vi "main.vi"() -> ()   [LabVIEW 2012]
uses:
  <vilib>/Instr/_visa.llb/VISA Configure Serial Port (Instr).vi
panel:
  in  "VISA":refnum<visa-resource-name>="COM6"
  in  "退出":bool
  in  "系统设置":bool
  in  "病例管理":bool
  in  "创建用户":bool
  in  "震动4":enum32{"选项卡 1", "选项卡 2"}(tab)
  in  "震动3":enum32{"选项卡 1", "选项卡 2"}(tab)
  in  "震动2":enum32{"选项卡 1", "选项卡 2"}(tab)
  in  "震动1":enum32{"选项卡 1", "选项卡 2"}(tab)
  in  "定频 4":T1=1 items=["定频1"=1, "定频2"=2, "定频3"=3, "定频4"=4, "定频5"=5, "定频6"=6, "定频7"=7, "定频8"=8, "定频9"=9]
  in  "变频 4":T2=1 items=["变频1"=1, "变频2"=2, "变频3"=3, "变频4"=4, "变频5"=5, "变频6"=6, "变频7"=7, "变频8"=8, "变频9"=9, "变频10"=10, "变频11"=11]
  in  "输出 4":T3
  in  "停止 4":T4
  in  "震动 4":T5
  in  "档位 4":T6
  in  "定时 4":T7=1800 items=["5分钟"=300, "10分钟"=600, "20分钟"=1200, "30分钟"=1800, "60分钟"=3600, "90分钟"=5400, "120分钟"=7200, "180分钟"=10800]
  out "time 4":T8
  in  "定频 3":T1=1 items=["定频1"=1, "定频2"=2, "定频3"=3, "定频4"=4, "定频5"=5, "定频6"=6, "定频7"=7, "定频8"=8, "定频9"=9]
  in  "变频 3":T2=1 items=["变频1"=1, "变频2"=2, "变频3"=3, "变频4"=4, "变频5"=5, "变频6"=6, "变频7"=7, "变频8"=8, "变频9"=9, "变频10"=10, "变频11"=11]
  in  "输出 3":T3
  in  "停止 3":T4
  in  "震动 3":T5
  in  "档位 3":T6
  in  "定时 3":T7=1800 items=["5分钟"=300, "10分钟"=600, "20分钟"=1200, "30分钟"=1800, "60分钟"=3600, "90分钟"=5400, "120分钟"=7200, "180分钟"=10800]
  out "time 3":T8
  in  "定频 2":T1=1 items=["定频1"=1, "定频2"=2, "定频3"=3, "定频4"=4, "定频5"=5, "定频6"=6, "定频7"=7, "定频8"=8, "定频9"=9]
  in  "变频 2":T2=1 items=["变频1"=1, "变频2"=2, "变频3"=3, "变频4"=4, "变频5"=5, "变频6"=6, "变频7"=7, "变频8"=8, "变频9"=9, "变频10"=10, "变频11"=11]
  in  "输出 2":T3
  in  "停止 2":T4
  in  "震动 2":T5
  in  "档位 2":T6
  in  "定时 2":T7=1800 items=["5分钟"=300, "10分钟"=600, "20分钟"=1200, "30分钟"=1800, "60分钟"=3600, "90分钟"=5400, "120分钟"=7200, "180分钟"=10800]
  out "time 2":T8
  in  "定频 1":T1=1 items=["定频1"=1, "定频2"=2, "定频3"=3, "定频4"=4, "定频5"=5, "定频6"=6, "定频7"=7, "定频8"=8, "定频9"=9]
  in  "变频 1":T2=1 items=["变频1"=1, "变频2"=2, "变频3"=3, "变频4"=4, "变频5"=5, "变频6"=6, "变频7"=7, "变频8"=8, "变频9"=9, "变频10"=10, "变频11"=11]
  in  "输出 1":T3
  in  "停止 1":T4
  in  "震动 1":T5
  in  "档位 1":T6
  in  "定时 1":T7=1800 items=["5分钟"=300, "10分钟"=600, "20分钟"=1200, "30分钟"=1800, "60分钟"=3600, "90分钟"=5400, "120分钟"=7200, "180分钟"=10800]
  out "time 1":T8
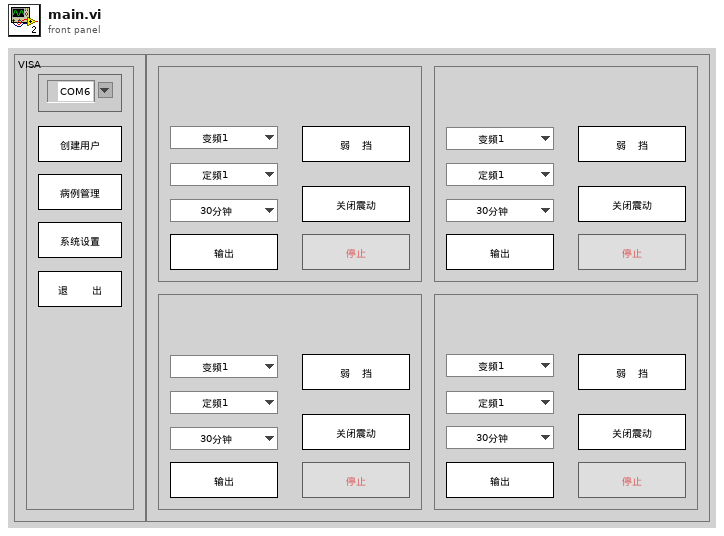
[diagram p1: front panel]
types:
  T1 = typedef "定频.ctl" = u8
  T2 = typedef "变频.ctl" = u8
  T3 = typedef "输出.ctl" = bool
  T4 = typedef "停止.ctl" = bool
  T5 = typedef "震动.ctl" = bool
  T6 = typedef "档位.ctl" = bool
  T7 = typedef "定时.ctl" = u16
  T8 = typedef "倒计时.ctl" = string
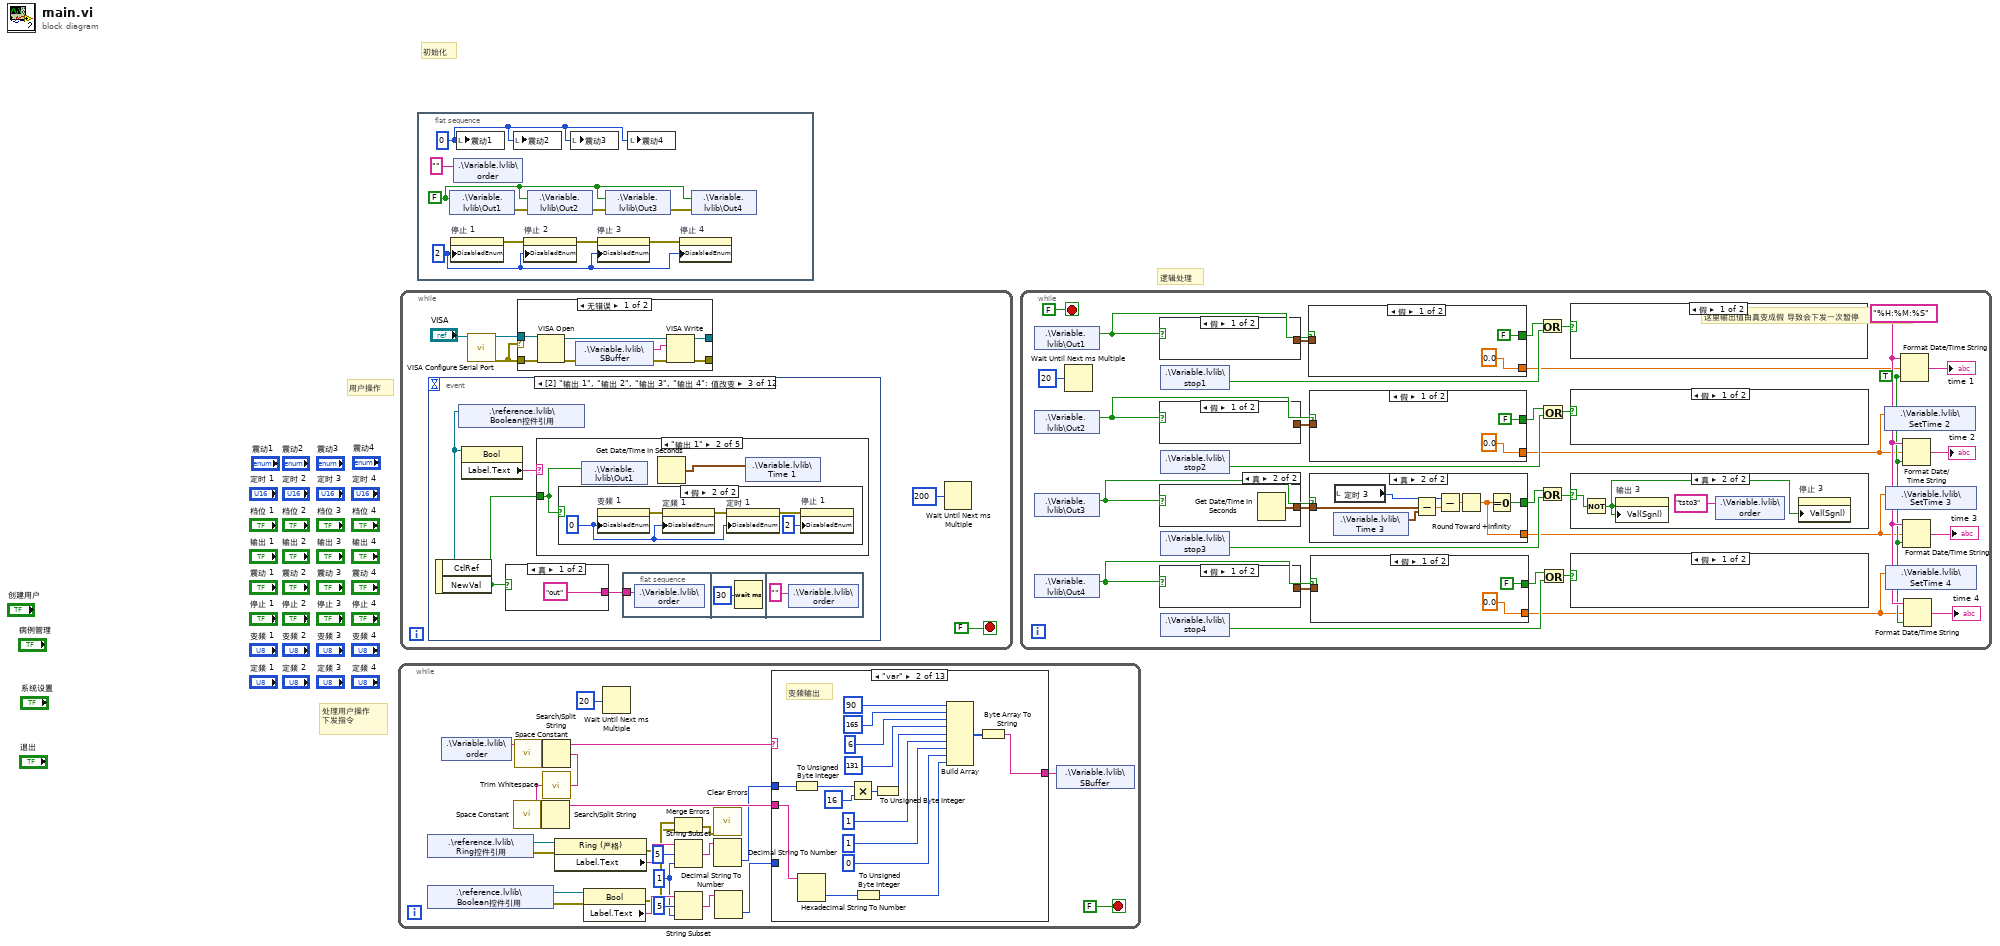
[diagram p0: block diagram]
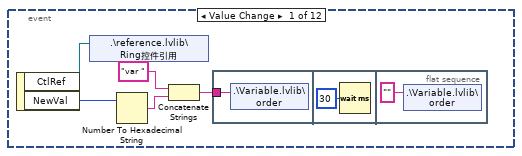
[diagram p3: hidden frame]
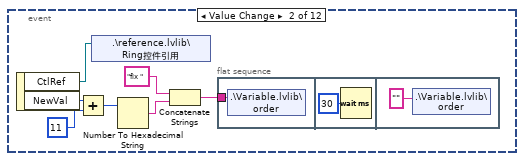
[diagram p4: hidden frame]
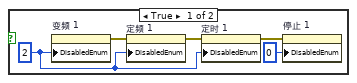
[diagram p6: hidden frame]
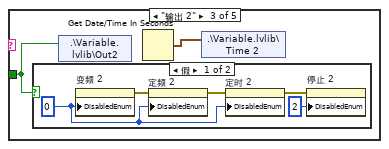
[diagram p7: hidden frame]
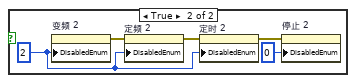
[diagram p8: hidden frame]
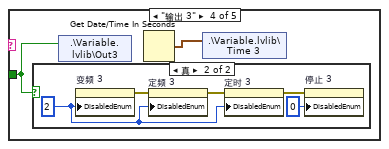
[diagram p9: hidden frame]
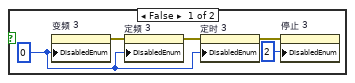
[diagram p10: hidden frame]
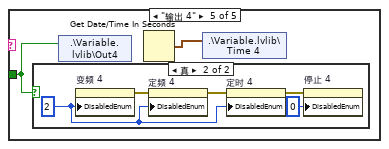
[diagram p11: hidden frame]
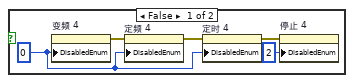
[diagram p12: hidden frame]
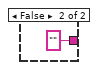
[diagram p13: hidden frame]
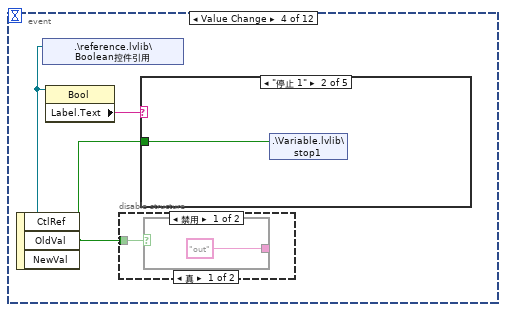
[diagram p14: hidden frame]
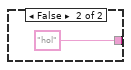
[diagram p15: hidden frame]
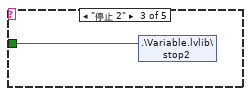
[diagram p18: hidden frame]
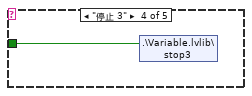
[diagram p19: hidden frame]
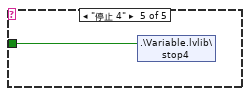
[diagram p20: hidden frame]
diagram:
  # "逻辑处理"
  # "处理用户操作\n下发指令"
  # "用户操作"
  # "初始化"
  # "这里输出值由真变成假 导致会下发一次暂停"
  n1 = while {
    stop <- FALSE stop-if-true
    w11 = 1
    n2 = shared-variable ".\\reference.lvlib\\Ring控件引用"() -> (w19:refnum<vi>, error out=w18:errorcluster)  [unwired: 1 in]
    n3 = shared-variable ".\\reference.lvlib\\Boolean控件引用"() -> (w17:refnum<vi>, error out=w16:errorcluster)  [unwired: 1 in]
    n4 = shared-variable ".\\Variable.lvlib\\order"() -> (w22:string)  [unwired: 1 in, 1 out]
    n5 = call <vilib>:"Space Constant.vi"() -> ("String"=w24:string)
    n6 = call <vilib>:"Space Constant.vi"() -> ("String"=w26:string)
    n7 = Search/Split String(string=w22, search string/char (-)=w26) -> (substring before match=w25:string, match + rest of string=w21:string)  [unwired: 1 in, 1 out]
    n8 = call <vilib>:"Trim Whitespace.vi"("string"=w21) -> ("trimmed string"=w20:string)  [unwired: 1 in]
    n9 = Search/Split String(string=w20, search string/char (-)=w24) -> (substring before match=w23:string)  [unwired: 1 in, 2 out]
    n10 = property class="Ring (严格)"(reference=w19, error in=w18) -> (error out=w5:errorcluster, "Label.Text"=w15:string)  [unwired: 1 out]
    n11 = property class="Bool"(reference=w17, error in=w16) -> (error out=w4:errorcluster, "Label.Text"=w13:string)  [unwired: 1 out]
    n12 = Wait Until Next ms Multiple(millisecond multiple=u32 20 ("毫秒倍数")) -> ()  [unwired: 1 out]
    n13 = Merge Errors(w5, w4) -> (w6:errorcluster)
    n14 = String Subset(string=w15, offset (0)=5 ("偏移量(0)"), length (rest)=w11) -> (substring=w10:string)
    n15 = String Subset(string=w13, offset (0)=5 ("偏移量(0)"), length (rest)=w11) -> (substring=w9:string)
    n16 = call <vilib>:"Clear Errors.vi"("error in (no error)"=w6) -> ()  [unwired: 6 in, 1 out]
    n17 = Decimal String To Number(string=w10) -> (number=w8:i32)  [unwired: 2 in, 1 out]
    n18 = Decimal String To Number(string=w9) -> (number=w7:i32)  [unwired: 2 in, 1 out]
    n19 = case shown="\"var\"" w25 {
      tunnel: w23 -> [_ w44 w61 _ _ _ _ _ _ _ _ _ _]
      tunnel: ["" ("string") w28 w45 w62 w77 w92 w106 w120 w134 w149 w168 w186 w201] -> w3
      tunnel: w8 -> [_ w30 w47 _ _ _ _ _ _ _ _ _ _]
      tunnel: w7 -> [_ _ _ w64 w79 _ _ _ _ w148 w167 w188 w203]
      frame Default {
      }
      frame "var" {
        # "变频输出"
        n20 = To Unsigned Byte Integer(number=w30) -> (unsigned 8bit integer=w29:u8)
        n21 = Hexadecimal String To Number(string=w44) -> (number=w36:u32)  [unwired: 2 in, 1 out]
        n22 = Multiply(x=w29, y=u8 16) -> (x*y=w37:u8)
        n23 = To Unsigned Byte Integer(number=w36) -> (unsigned 8bit integer=w31:u8)
        n24 = To Unsigned Byte Integer(number=w37) -> (unsigned 8bit integer=w35:u8)
        n25 = Build Array(u8 90, u8 165, u8 6, u8 131, w35, u8 1, u8 1, u8 0, w31) -> (w42:u8[])
        n26 = Byte Array To String(unsigned byte array=w42) -> (string=w28:string)
      }
      frame "fix" {
        # "定频输出"
        n27 = To Unsigned Byte Integer(number=w47) -> (unsigned 8bit integer=w46:u8)
        n28 = Hexadecimal String To Number(string=w61) -> (number=w53:u32)  [unwired: 2 in, 1 out]
        n29 = Multiply(x=w46, y=u8 16) -> (x*y=w54:u8)
        n30 = To Unsigned Byte Integer(number=w53) -> (unsigned 8bit integer=w48:u8)
        n31 = To Unsigned Byte Integer(number=w54) -> (unsigned 8bit integer=w52:u8)
        n32 = Build Array(u8 90, u8 165, u8 6, u8 131, w52, u8 1, u8 1, u8 0, w48) -> (w59:u8[])
        n33 = Byte Array To String(unsigned byte array=w59) -> (string=w45:string)
      }
      frame "out" {
        # "输出"
        n34 = To Unsigned Byte Integer(number=w64) -> (unsigned 8bit integer=w63:u8)
        n35 = Multiply(x=w63, y=u8 16) -> (x*y=w70:u8)
        n36 = To Unsigned Byte Integer(number=w70) -> (unsigned 8bit integer=w69:u8)
        n37 = Build Array(u8 90, u8 165, u8 6, u8 131, w69, u8 0, u8 1, u8 0, u8 1) -> (w75:u8[])
        n38 = Byte Array To String(unsigned byte array=w75) -> (string=w62:string)
      }
      frame "sto" {
        n39 = To Unsigned Byte Integer(number=w79) -> (unsigned 8bit integer=w78:u8)
        n40 = Multiply(x=w78, y=u8 16) -> (x*y=w85:u8)
        n41 = To Unsigned Byte Integer(number=w85) -> (unsigned 8bit integer=w84:u8)
        n42 = Build Array(u8 90, u8 165, u8 6, u8 131, w84, u8 0, u8 1, u8 0, u8 0) -> (w90:u8[])
        n43 = Byte Array To String(unsigned byte array=w90) -> (string=w77:string)
      }
      frame "tsto1" {
        n44 = Multiply(x=u8 1, y=u8 16) -> (x*y=w99:u8)
        n45 = To Unsigned Byte Integer(number=w99) -> (unsigned 8bit integer=w98:u8)
        n46 = Build Array(u8 90, u8 165, u8 6, u8 131, w98, u8 0, u8 1, u8 0, u8 0) -> (w104:u8[])
        n47 = Byte Array To String(unsigned byte array=w104) -> (string=w92:string)
      }
      frame "tsto2" {
        n48 = Multiply(x=u8 2, y=u8 16) -> (x*y=w113:u8)
        n49 = To Unsigned Byte Integer(number=w113) -> (unsigned 8bit integer=w112:u8)
        n50 = Build Array(u8 90, u8 165, u8 6, u8 131, w112, u8 0, u8 1, u8 0, u8 0) -> (w118:u8[])
        n51 = Byte Array To String(unsigned byte array=w118) -> (string=w106:string)
      }
      frame "tsto3" {
        n52 = Multiply(x=u8 3, y=u8 16) -> (x*y=w127:u8)
        n53 = To Unsigned Byte Integer(number=w127) -> (unsigned 8bit integer=w126:u8)
        n54 = Build Array(u8 90, u8 165, u8 6, u8 131, w126, u8 0, u8 1, u8 0, u8 0) -> (w132:u8[])
        n55 = Byte Array To String(unsigned byte array=w132) -> (string=w120:string)
      }
      frame "tsto4" {
        n56 = Multiply(x=u8 4, y=u8 16) -> (x*y=w141:u8)
        n57 = To Unsigned Byte Integer(number=w141) -> (unsigned 8bit integer=w140:u8)
        n58 = Build Array(u8 90, u8 165, u8 6, u8 131, w140, u8 0, u8 1, u8 0, u8 0) -> (w146:u8[])
        n59 = Byte Array To String(unsigned byte array=w146) -> (string=w134:string)
      }
      frame "sha" {
        n60 = To Unsigned Byte Integer(number=w148) -> (unsigned 8bit integer=w150:u8)
        n61 = Multiply(x=w150, y=u8 16) -> (x*y=w156:u8)
        n62 = To Unsigned Byte Integer(number=w156) -> (unsigned 8bit integer=w155:u8)
        n63 = Build Array(u8 90, u8 165, u8 6, u8 131, w155, u8 6, u8 1, u8 0, u8 1) -> (w161:u8[])
        n64 = case shown="4" w148 {
          frame 0, Default {
          }
          frame 1 {
            n65 = local write "震动1"(0) -> ()
          }
          frame 2 {
            n66 = local write "震动2"(0) -> ()
          }
          frame 3 {
            n67 = local write "震动3"(0) -> ()
          }
          frame 4 {
            n68 = local write "震动4"(0) -> ()
          }
        }
        n69 = Byte Array To String(unsigned byte array=w161) -> (string=w149:string)
      }
      frame "sth" {
        n70 = To Unsigned Byte Integer(number=w167) -> (unsigned 8bit integer=w169:u8)
        n71 = Multiply(x=w169, y=u8 16) -> (x*y=w175:u8)
        n72 = To Unsigned Byte Integer(number=w175) -> (unsigned 8bit integer=w174:u8)
        n73 = Build Array(u8 90, u8 165, u8 6, u8 131, w174, u8 6, u8 1, u8 0, u8 0) -> (w180:u8[])
        n74 = case shown="0, 默认" w167 {
          frame 0, Default {
          }
          frame 1 {
            n75 = local write "震动1"(1) -> ()
          }
          frame 2 {
            n76 = local write "震动2"(1) -> ()
          }
          frame 3 {
            n77 = local write "震动3"(1) -> ()
          }
          frame 4 {
            n78 = local write "震动4"(1) -> ()
          }
        }
        n79 = Byte Array To String(unsigned byte array=w180) -> (string=w168:string)
      }
      frame "pw1" {
        n80 = To Unsigned Byte Integer(number=w188) -> (unsigned 8bit integer=w187:u8)
        n81 = Multiply(x=w187, y=u8 16) -> (x*y=w194:u8)
        n82 = To Unsigned Byte Integer(number=w194) -> (unsigned 8bit integer=w193:u8)
        n83 = Build Array(u8 90, u8 165, u8 6, u8 131, w193, u8 5, u8 1, u8 0, u8 0) -> (w199:u8[])
        n84 = Byte Array To String(unsigned byte array=w199) -> (string=w186:string)
      }
      frame "pw2" {
        n85 = To Unsigned Byte Integer(number=w203) -> (unsigned 8bit integer=w202:u8)
        n86 = Multiply(x=w202, y=u8 16) -> (x*y=w209:u8)
        n87 = To Unsigned Byte Integer(number=w209) -> (unsigned 8bit integer=w208:u8)
        n88 = Build Array(u8 90, u8 165, u8 6, u8 131, w208, u8 5, u8 1, u8 0, u8 1) -> (w214:u8[])
        n89 = Byte Array To String(unsigned byte array=w214) -> (string=w201:string)
      }
    }
    n90 = shared-variable ".\\Variable.lvlib\\SBuffer"(w3) -> ()  [unwired: 1 in, 1 out]
  }
  n91 = while {
    stop <- FALSE stop-if-true
    n92 = event shown="[2] \"输出 1\", \"输出 2\", \"输出 3\", \"输出 4\": 值改变" {
      selector: _ -> [_ _ _ _ _ _ _ _ _ _ _ _]
      dyn-events: _ -> [_ _ _ _ _ _ _ _ _ _ _ _]
      timeout: _ -> [_ _ _ _ _ _ _ _ _ _ _ _]
      event Value Change {
        n93 = event-data() -> ("CtlRef"=w232:refnum<vi>, "NewVal"=w233:T2)  [unwired: 1 in]
        n94 = shared-variable ".\\reference.lvlib\\Ring控件引用"(w232) -> ()  [unwired: 1 in, 1 out]
        n95 = Number To Hexadecimal String(2:w233) -> (0:w235:string)  [unwired: 1 in]
        n96 = Concatenate Strings("var " ("字符串"), w235) -> (w231:string)
        n97 = flat-sequence {
          tunnel: w231 -> [w236]
          frame #0 {
            n98 = shared-variable ".\\Variable.lvlib\\order"(w236) -> ()  [unwired: 1 in, 1 out]
          }
          frame #1 {
            n99 = Wait (ms)(milliseconds to wait=u32 30 ("等待时间（毫秒）")) -> ()  [unwired: 1 out]
          }
          frame #2 {
            n100 = shared-variable ".\\Variable.lvlib\\order"("" ("order")) -> ()  [unwired: 1 in, 1 out]
          }
        }
      }
      event Value Change {
        n101 = event-data() -> ("CtlRef"=w240:refnum<vi>, "NewVal"=w242:T1)  [unwired: 1 in]
        n102 = Add(x=w242, y=11) -> (x+y=w243:i32)
        n103 = shared-variable ".\\reference.lvlib\\Ring控件引用"(w240) -> ()  [unwired: 1 in, 1 out]
        n104 = Number To Hexadecimal String(2:w243) -> (0:w245:string)  [unwired: 1 in]
        n105 = Concatenate Strings("fix " ("字符串"), w245) -> (w239:string)
        n106 = flat-sequence {
          tunnel: w239 -> [w246]
          frame #0 {
            n107 = shared-variable ".\\Variable.lvlib\\order"(w246) -> ()  [unwired: 1 in, 1 out]
          }
          frame #1 {
            n108 = Wait (ms)(milliseconds to wait=u32 30 ("等待时间（毫秒）")) -> ()  [unwired: 1 out]
          }
          frame #2 {
            n109 = shared-variable ".\\Variable.lvlib\\order"("" ("order")) -> ()  [unwired: 1 in, 1 out]
          }
        }
      }
      event Value Change {
        n110 = event-data() -> ("CtlRef"=w250:refnum<vi>, "NewVal"=w251:T3)  [unwired: 1 in]
        n111 = shared-variable ".\\reference.lvlib\\Boolean控件引用"(w250) -> ()  [unwired: 1 in, 1 out]
        n112 = property class="Bool"(reference=w250) -> ("Label.Text"=w252:string)  [unwired: 1 in, 2 out]
        n113 = case shown="真" w251 {
          tunnel: ["out" ""] -> w249
          frame True {
          }
          frame False {
          }
        }
        n114 = case shown="\"输出 1\"" w252 {
          tunnel: w251 -> [_ w257 w269 w281 w293]
          frame "假", Default {
          }
          frame "输出 1" {
            n115 = case shown="假" w257 {
              frame True {
                w259 = 2
                n116 = property on="变频 1" class="Ring (严格)"("DisabledEnum"=w259) -> (error out=w262:errorcluster)  [unwired: 2 in, 1 out]
                n117 = property on="定频 1" class="Ring (严格)"(error in=w262, "DisabledEnum"=w259) -> (error out=w261:errorcluster)  [unwired: 1 in, 1 out]
                n118 = property on="定时 1" class="Ring (严格)"(error in=w261, "DisabledEnum"=w259) -> (error out=w260:errorcluster)  [unwired: 1 in, 1 out]
                n119 = property on="停止 1" class="Bool"(error in=w260, "DisabledEnum"=0) -> ()  [unwired: 1 in, 2 out]
              }
              frame False {
                w264 = 0
                n120 = property on="变频 1" class="Ring (严格)"("DisabledEnum"=w264) -> (error out=w267:errorcluster)  [unwired: 2 in, 1 out]
                n121 = property on="定频 1" class="Ring (严格)"(error in=w267, "DisabledEnum"=w264) -> (error out=w266:errorcluster)  [unwired: 1 in, 1 out]
                n122 = property on="定时 1" class="Ring (严格)"(error in=w266, "DisabledEnum"=w264) -> (error out=w265:errorcluster)  [unwired: 1 in, 1 out]
                n123 = property on="停止 1" class="Bool"(error in=w265, "DisabledEnum"=2) -> ()  [unwired: 1 in, 2 out]
              }
            }
            n124 = shared-variable ".\\Variable.lvlib\\Out1"(w257) -> ()  [unwired: 1 in, 1 out]
            n125 = Get Date/Time In Seconds() -> (seconds since 1Jan1904=w256:timestamp)
            n126 = shared-variable ".\\Variable.lvlib\\Time 1"(w256) -> ()  [unwired: 1 in, 1 out]
          }
          frame "输出 2" {
            n127 = case shown="假" w269 {
              frame False {
                w271 = 0
                n128 = property on="变频 2" class="Ring (严格)"("DisabledEnum"=w271) -> (error out=w274:errorcluster)  [unwired: 2 in, 1 out]
                n129 = property on="定频 2" class="Ring (严格)"(error in=w274, "DisabledEnum"=w271) -> (error out=w273:errorcluster)  [unwired: 1 in, 1 out]
                n130 = property on="定时 2" class="Ring (严格)"(error in=w273, "DisabledEnum"=w271) -> (error out=w272:errorcluster)  [unwired: 1 in, 1 out]
                n131 = property on="停止 2" class="Bool"(error in=w272, "DisabledEnum"=2) -> ()  [unwired: 1 in, 2 out]
              }
              frame True {
                w276 = 2
                n132 = property on="变频 2" class="Ring (严格)"("DisabledEnum"=w276) -> (error out=w279:errorcluster)  [unwired: 2 in, 1 out]
                n133 = property on="定频 2" class="Ring (严格)"(error in=w279, "DisabledEnum"=w276) -> (error out=w278:errorcluster)  [unwired: 1 in, 1 out]
                n134 = property on="定时 2" class="Ring (严格)"(error in=w278, "DisabledEnum"=w276) -> (error out=w277:errorcluster)  [unwired: 1 in, 1 out]
                n135 = property on="停止 2" class="Bool"(error in=w277, "DisabledEnum"=0) -> ()  [unwired: 1 in, 2 out]
              }
            }
            n136 = shared-variable ".\\Variable.lvlib\\Out2"(w269) -> ()  [unwired: 1 in, 1 out]
            n137 = Get Date/Time In Seconds() -> (seconds since 1Jan1904=w268:timestamp)
            n138 = shared-variable ".\\Variable.lvlib\\Time 2"(w268) -> ()  [unwired: 1 in, 1 out]
          }
          frame "输出 3" {
            n139 = case shown="真" w281 {
              frame False {
                w283 = 0
                n140 = property on="变频 3" class="Ring (严格)"("DisabledEnum"=w283) -> (error out=w286:errorcluster)  [unwired: 2 in, 1 out]
                n141 = property on="定频 3" class="Ring (严格)"(error in=w286, "DisabledEnum"=w283) -> (error out=w285:errorcluster)  [unwired: 1 in, 1 out]
                n142 = property on="定时 3" class="Ring (严格)"(error in=w285, "DisabledEnum"=w283) -> (error out=w284:errorcluster)  [unwired: 1 in, 1 out]
                n143 = property on="停止 3" class="Bool"(error in=w284, "DisabledEnum"=2) -> ()  [unwired: 1 in, 2 out]
              }
              frame True {
                w288 = 2
                n144 = property on="变频 3" class="Ring (严格)"("DisabledEnum"=w288) -> (error out=w291:errorcluster)  [unwired: 2 in, 1 out]
                n145 = property on="定频 3" class="Ring (严格)"(error in=w291, "DisabledEnum"=w288) -> (error out=w290:errorcluster)  [unwired: 1 in, 1 out]
                n146 = property on="定时 3" class="Ring (严格)"(error in=w290, "DisabledEnum"=w288) -> (error out=w289:errorcluster)  [unwired: 1 in, 1 out]
                n147 = property on="停止 3" class="Bool"(error in=w289, "DisabledEnum"=0) -> ()  [unwired: 1 in, 2 out]
              }
            }
            n148 = shared-variable ".\\Variable.lvlib\\Out3"(w281) -> ()  [unwired: 1 in, 1 out]
            n149 = Get Date/Time In Seconds() -> (seconds since 1Jan1904=w280:timestamp)
            n150 = shared-variable ".\\Variable.lvlib\\Time 3"(w280) -> ()  [unwired: 1 in, 1 out]
          }
          frame "输出 4" {
            n151 = case shown="真" w293 {
              frame False {
                w295 = 0
                n152 = property on="变频 4" class="Ring (严格)"("DisabledEnum"=w295) -> (error out=w298:errorcluster)  [unwired: 2 in, 1 out]
                n153 = property on="定频 4" class="Ring (严格)"(error in=w298, "DisabledEnum"=w295) -> (error out=w297:errorcluster)  [unwired: 1 in, 1 out]
                n154 = property on="定时 4" class="Ring (严格)"(error in=w297, "DisabledEnum"=w295) -> (error out=w296:errorcluster)  [unwired: 1 in, 1 out]
                n155 = property on="停止 4" class="Bool"(error in=w296, "DisabledEnum"=2) -> ()  [unwired: 1 in, 2 out]
              }
              frame True {
                w300 = 2
                n156 = property on="变频 4" class="Ring (严格)"("DisabledEnum"=w300) -> (error out=w303:errorcluster)  [unwired: 2 in, 1 out]
                n157 = property on="定频 4" class="Ring (严格)"(error in=w303, "DisabledEnum"=w300) -> (error out=w302:errorcluster)  [unwired: 1 in, 1 out]
                n158 = property on="定时 4" class="Ring (严格)"(error in=w302, "DisabledEnum"=w300) -> (error out=w301:errorcluster)  [unwired: 1 in, 1 out]
                n159 = property on="停止 4" class="Bool"(error in=w301, "DisabledEnum"=0) -> ()  [unwired: 1 in, 2 out]
              }
            }
            n160 = shared-variable ".\\Variable.lvlib\\Out4"(w293) -> ()  [unwired: 1 in, 1 out]
            n161 = Get Date/Time In Seconds() -> (seconds since 1Jan1904=w292:timestamp)
            n162 = shared-variable ".\\Variable.lvlib\\Time 4"(w292) -> ()  [unwired: 1 in, 1 out]
          }
        }
        n163 = flat-sequence {
          tunnel: w249 -> [w253]
          frame #0 {
            n164 = shared-variable ".\\Variable.lvlib\\order"(w253) -> ()  [unwired: 1 in, 1 out]
          }
          frame #1 {
            n165 = Wait (ms)(milliseconds to wait=u32 30 ("等待时间（毫秒）")) -> ()  [unwired: 1 out]
          }
          frame #2 {
            n166 = shared-variable ".\\Variable.lvlib\\order"("" ("order")) -> ()  [unwired: 1 in, 1 out]
          }
        }
      }
      event Value Change {
        n167 = event-data() -> ("CtlRef"=w307:refnum<vi>, "NewVal"=w306:T4)  [unwired: 1 in, 1 out]
        n168 = shared-variable ".\\reference.lvlib\\Boolean控件引用"(w307) -> ()  [unwired: 1 in, 1 out]
        n169 = property class="Bool"(reference=w307) -> ("Label.Text"=w308:string)  [unwired: 1 in, 2 out]
        n170 = disable-structure shown="禁用" {
          disable-tunnel: w306 -> [w309 _]
          frame Disabled {
            n171 = case shown="真" w309 {
              tunnel: ["out" "hol"] -> _
              frame True {
              }
              frame False {
              }
            }
          }
          frame Enabled {
          }
        }
        n172 = case shown="\"停止 1\"" w308 {
          tunnel: w306 -> [_ w312 w313 w314 w315]
          frame "假", Default {
          }
          frame "停止 1" {
            n173 = shared-variable ".\\Variable.lvlib\\stop1"(w312) -> ()  [unwired: 1 in, 1 out]
          }
          frame "停止 2" {
            n174 = shared-variable ".\\Variable.lvlib\\stop2"(w313) -> ()  [unwired: 1 in, 1 out]
          }
          frame "停止 3" {
            n175 = shared-variable ".\\Variable.lvlib\\stop3"(w314) -> ()  [unwired: 1 in, 1 out]
          }
          frame "停止 4" {
            n176 = shared-variable ".\\Variable.lvlib\\stop4"(w315) -> ()  [unwired: 1 in, 1 out]
          }
        }
      }
      event Value Change {
        n177 = event-data() -> ("CtlRef"=w316:refnum<vi>, "NewVal"=w318:T5)  [unwired: 1 in]
        n178 = shared-variable ".\\reference.lvlib\\Boolean控件引用"(w316) -> ()  [unwired: 1 in, 1 out]
        n179 = case shown="真" w318 {
          tunnel: ["sth" "sha"] -> w317
          frame True {
          }
          frame False {
          }
        }
        n180 = flat-sequence {
          tunnel: w317 -> [w319]
          frame #0 {
            n181 = shared-variable ".\\Variable.lvlib\\order"(w319) -> ()  [unwired: 1 in, 1 out]
          }
          frame #1 {
            n182 = Wait (ms)(milliseconds to wait=u32 30 ("等待时间（毫秒）")) -> ()  [unwired: 1 out]
          }
          frame #2 {
            n183 = shared-variable ".\\Variable.lvlib\\order"("" ("order")) -> ()  [unwired: 1 in, 1 out]
          }
        }
      }
      event Value Change {
        n184 = event-data() -> ("CtlRef"=w325:refnum<vi>, "NewVal"=w326:T6)  [unwired: 1 in]
        n185 = shared-variable ".\\reference.lvlib\\Boolean控件引用"(w325) -> ()  [unwired: 1 in, 1 out]
        n186 = case shown="假" w326 {
          tunnel: ["pw2" "pw1"] -> w324
          frame True {
          }
          frame False {
          }
        }
        n187 = flat-sequence {
          tunnel: w324 -> [w327]
          frame #0 {
            n188 = shared-variable ".\\Variable.lvlib\\order"(w327) -> ()  [unwired: 1 in, 1 out]
          }
          frame #1 {
            n189 = Wait (ms)(milliseconds to wait=u32 30 ("等待时间（毫秒）")) -> ()  [unwired: 1 out]
          }
          frame #2 {
            n190 = shared-variable ".\\Variable.lvlib\\order"("" ("order")) -> ()  [unwired: 1 in, 1 out]
          }
        }
      }
      event "VISA": Value Change {
        n191 = event-data() -> ("OldVal"=w335:refnum<visa-resource-name>, "NewVal"=w334:refnum<visa-resource-name>)  [unwired: 1 in]
        n192 = VISA Close(VISA resource name=w335) -> (error out=w333:errorcluster)  [unwired: 1 in]
        n193 = VISA Open(error in (no error)=w333, VISA resource name=w334) -> (error out=w332:errorcluster)  [unwired: 3 in, 1 out]
        n194 = call <vilib>:"General Error Handler.vi"("error in (no error)"=w332) -> ()  [unwired: 10 in, 5 out]
      }
      event Panel Close? {
        n195 = event-data() -> ()  [unwired: 1 in, 1 out]
        n196 = shared-variable ".\\Variable.lvlib\\Out4"() -> (w338:bool)  [unwired: 1 in, 1 out]
        n197 = shared-variable ".\\Variable.lvlib\\Out3"() -> (w339:bool)  [unwired: 1 in, 1 out]
        n198 = shared-variable ".\\Variable.lvlib\\Out1"() -> (w340:bool)  [unwired: 1 in, 1 out]
        n199 = shared-variable ".\\Variable.lvlib\\Out2"() -> (w341:bool)  [unwired: 1 in, 1 out]
        n200 = Compound Arithmetic op=OR(w340, w341, w339, w338) -> (w337:bool)
        n201 = case shown="假" w337 {
          tunnel: [w342 w345] -> w336
          frame True {
            n202 = Two Button Dialog(message="正在治疗中！！   \n请确认是否关闭" ("消息")) -> (T button?=w343:bool)  [unwired: 2 in]
            n203 = Not(x=w343) -> (.not. x?=w342:bool)
          }
          frame False {
            n204 = Two Button Dialog(message="软件即将关闭！" ("消息")) -> (T button?=w346:bool)  [unwired: 2 in]
            n205 = Not(x=w346) -> (.not. x?=w345:bool)
          }
        }
        n206 = event-data("Discard?"=w336) -> ()  [unwired: 1 in, 1 out]
      }
      event "退出": Value Change {
        n207 = event-data() -> ()  [unwired: 1 in, 3 out]
        n208 = shared-variable ".\\Variable.lvlib\\Out4"() -> (w350:bool)  [unwired: 1 in, 1 out]
        n209 = shared-variable ".\\Variable.lvlib\\Out3"() -> (w351:bool)  [unwired: 1 in, 1 out]
        n210 = shared-variable ".\\Variable.lvlib\\Out1"() -> (w352:bool)  [unwired: 1 in, 1 out]
        n211 = shared-variable ".\\Variable.lvlib\\Out2"() -> (w353:bool)  [unwired: 1 in, 1 out]
        n212 = Compound Arithmetic op=OR(w352, w353, w351, w350) -> (w349:bool)
        n213 = case shown="假" w349 {
          tunnel: [w355 w358] -> w348
          frame True {
            n214 = Two Button Dialog(message="正在治疗中！！   \n请确认是否关闭" ("消息")) -> (T button?=w356:bool)  [unwired: 2 in]
            n215 = Not(x=w356) -> (.not. x?=w355:bool)
          }
          frame False {
            n216 = Two Button Dialog(message="软件即将关闭！" ("消息")) -> (T button?=w358:bool)  [unwired: 2 in]
          }
        }
        n217 = case shown="真" w348 {
          frame False {
          }
          frame True {
            n218 = local read "VISA"() -> (w354:refnum<visa-resource-name>)
            n219 = VISA Close(VISA resource name=w354) -> ()  [unwired: 1 in, 1 out]
          }
        }
        n220 = Quit LabVIEW(quit? (T)=w348) -> ()
      }
      event "创建用户": Value Change {
        n221 = event-data() -> ()  [unwired: 1 in, 3 out]
        n222 = Current VI's Path() -> (path=w370:path)
        n223 = Build Path(base path=w370, name or relative path="..\\SubVIs\\adduser.vi" ("名称或相对路径")) -> (appended path=w371:path)
        n224 = Open VI Reference(vi path=w371) -> (vi reference=w368:refnum<vi>, error out=w367:errorcluster)  [unwired: 5 in]
        n225 = invoke class="VI" method="Run VI"(reference=w368, error in=w367, "Wait until done"=FALSE ("结束前等待"), "Auto Dispose Ref"=FALSE ("自动销毁引用")) -> (reference out=w364:refnum<vi>, error out=w363:errorcluster)  [unwired: 1 in, 3 out]
        n226 = invoke class="VI" method="FP.Open"(reference=w364, error in=w363, "Activate"=TRUE ("激活？")) -> (reference out=w360:refnum<vi>, error out=w361:errorcluster)  [unwired: 2 in, 3 out]
        n227 = Close Reference(reference=w360, error in (no error)=w361) -> ()  [unwired: 1 out]
      }
      event "病例管理": Value Change {
        n228 = event-data() -> ()  [unwired: 1 in, 3 out]
        n229 = Current VI's Path() -> (path=w383:path)
        n230 = Build Path(base path=w383, name or relative path="..\\SubVIs\\PatManage.vi" ("名称或相对路径")) -> (appended path=w384:path)
        n231 = Open VI Reference(vi path=w384) -> (vi reference=w381:refnum<vi>, error out=w380:errorcluster)  [unwired: 5 in]
        n232 = invoke class="VI" method="Run VI"(reference=w381, error in=w380, "Wait until done"=FALSE ("结束前等待"), "Auto Dispose Ref"=FALSE ("自动销毁引用")) -> (reference out=w377:refnum<vi>, error out=w376:errorcluster)  [unwired: 1 in, 3 out]
        n233 = invoke class="VI" method="FP.Open"(reference=w377, error in=w376, "Activate"=TRUE ("激活？")) -> (reference out=w373:refnum<vi>, error out=w374:errorcluster)  [unwired: 2 in, 3 out]
        n234 = Close Reference(reference=w373, error in (no error)=w374) -> (error out=w372:errorcluster)
        n235 = call <vilib>:"Clear Errors.vi"("error in (no error)"=w372) -> ()  [unwired: 6 in, 1 out]
      }
      event "系统设置": Value Change {
        n236 = event-data() -> ()  [unwired: 1 in, 3 out]
        n237 = call "医院信息设置"() -> ("联系电话"=w390:string, "联系人"=w391:string, "医院地址"=w392:string, "医院名称"=w393:string, "确定"=w385:bool)  [unwired: 14 in, 1 out]
        n238 = Current VI's Path() -> (path=w397:path)
        n239 = case shown="假" w385 {
          tunnel: w393 -> [_ w404]
          tunnel: w392 -> [_ w403]
          tunnel: w391 -> [_ w402]
          tunnel: w390 -> [_ w400]
          tunnel: [_ w399] -> w389
          frame False {
          }
          frame True {
            n240 = call <vilib>:"Space Constant.vi"() -> ("String"=w401:string)
            n241 = Concatenate Strings(w404, w401, w403, w401, w402, w401, w400) -> (w399:string)
          }
        }
        n242 = Build Path(base path=w397, name or relative path="..\\DATA\\HosInfor.txt" ("名称或相对路径")) -> (appended path=w398:path)
        n243 = Open/Create/Replace File(file path (use dialog)=w398) -> (refnum out=w394:refnum<file>, error out=w395:errorcluster)  [unwired: 5 in, 1 out]
        n244 = Write to Text File(file (use dialog)=w394, text=w389, error in=w395) -> (refnum out=w388:refnum<file>, error out=w386:errorcluster)  [unwired: 1 in, 1 out]
        n245 = case shown="真" w385 {
          tunnel: w386 -> [_ w405]
          frame False {
          }
          frame True {
            n246 = case shown="无错误" w405 {
              frame No Error {
                n247 = One Button Dialog(message="设置成功！" ("消息")) -> ()  [unwired: 1 in, 1 out]
              }
              frame Error {
              }
            }
          }
        }
        n248 = Close File(refnum=w388, error in=w386) -> (error out=w387:errorcluster)  [unwired: 1 out]
        n249 = call <vilib>:"General Error Handler.vi"("error in (no error)"=w387) -> ()  [unwired: 10 in, 5 out]
      }
    }
    n250 = call-poly "VISA Configure Serial Port"("VISA resource name"="VISA") -> ("VISA resource name out"=w219:refnum<visa-resource-name>, "error out"=w218:errorcluster)  [unwired: 13 in]
    n251 = case shown="无错误" w218 {
      tunnel: w219 -> [w223 w230]
      tunnel: w218 -> [w221 w229]
      tunnel: [w228 w229] -> _
      tunnel: [w227 w230] -> _
      frame No Error {
        n252 = VISA Open(error in (no error)=w221, VISA resource name=w223) -> (VISA resource name=w222:refnum<visa-resource-name>, error out=w224:errorcluster)  [unwired: 3 in]
        n253 = shared-variable ".\\Variable.lvlib\\SBuffer"(error in=w224) -> (w225:string, error out=w226:errorcluster)
        n254 = VISA Write(VISA resource name=w222, write buffer=w225, error in (no error)=w226) -> (VISA resource name out=w227:refnum<visa-resource-name>, error out=w228:errorcluster)  [unwired: 1 out]
      }
      frame Error {
      }
    }
    n255 = Wait Until Next ms Multiple(millisecond multiple=u32 200 ("毫秒倍数")) -> ()  [unwired: 1 out]
  }
  n256 = flat-sequence {
    frame #0 {
      w407 = 0
      w409 = FALSE ("Out1")
      w413 = 2
      n257 = shared-variable ".\\Variable.lvlib\\Out1"(w409) -> (error out=w412:errorcluster)  [unwired: 1 in]
      n258 = property on="停止 1" class="Bool"("DisabledEnum"=w413) -> (error out=w416:errorcluster)  [unwired: 2 in, 1 out]
      n259 = shared-variable ".\\Variable.lvlib\\order"("" ("发送")) -> ()  [unwired: 1 in, 1 out]
      n260 = local write "震动1"(w407) -> ()
      n261 = local write "震动2"(w407) -> ()
      n262 = property on="停止 2" class="Bool"(error in=w416, "DisabledEnum"=w413) -> (error out=w415:errorcluster)  [unwired: 1 in, 1 out]
      n263 = shared-variable ".\\Variable.lvlib\\Out2"(w409, error in=w412) -> (error out=w411:errorcluster)
      n264 = local write "震动3"(w407) -> ()
      n265 = property on="停止 3" class="Bool"(error in=w415, "DisabledEnum"=w413) -> (error out=w414:errorcluster)  [unwired: 1 in, 1 out]
      n266 = shared-variable ".\\Variable.lvlib\\Out3"(w409, error in=w411) -> (error out=w410:errorcluster)
      n267 = local write "震动4"(w407) -> ()
      n268 = property on="停止 4" class="Bool"(error in=w414, "DisabledEnum"=w413) -> ()  [unwired: 1 in, 2 out]
      n269 = shared-variable ".\\Variable.lvlib\\Out4"(w409, error in=w410) -> ()  [unwired: 1 out]
    }
  }
  n270 = while {
    stop <- FALSE stop-if-true
    w434 = TRUE ("UTC格式")
    w439 = "%H:%M:%S" ("时间格式字符串(%c)")
    n271 = shared-variable ".\\Variable.lvlib\\Out1"() -> (w443:bool)  [unwired: 1 in, 1 out]
    n272 = shared-variable ".\\Variable.lvlib\\Out2"() -> (w442:bool)  [unwired: 1 in, 1 out]
    n273 = shared-variable ".\\Variable.lvlib\\Out3"() -> (w441:bool)  [unwired: 1 in, 1 out]
    n274 = shared-variable ".\\Variable.lvlib\\Out4"() -> (w440:bool)  [unwired: 1 in, 1 out]
    n275 = Wait Until Next ms Multiple(millisecond multiple=u32 20 ("毫秒倍数")) -> ()  [unwired: 1 out]
    n276 = case shown="假" w443 {
      tunnel: [_ w500] -> w447
      frame False {
      }
      frame True {
        n277 = Get Date/Time In Seconds() -> (seconds since 1Jan1904=w500:timestamp)
      }
    }
    n278 = case shown="假" w442 {
      tunnel: [_ w499] -> w446
      frame False {
      }
      frame True {
        n279 = Get Date/Time In Seconds() -> (seconds since 1Jan1904=w499:timestamp)
      }
    }
    n280 = case shown="真" w441 {
      tunnel: [_ w498] -> w445
      frame False {
      }
      frame True {
        n281 = Get Date/Time In Seconds() -> (seconds since 1Jan1904=w498:timestamp)
      }
    }
    n282 = case shown="假" w440 {
      tunnel: [_ w497] -> w444
      frame False {
      }
      frame True {
        n283 = Get Date/Time In Seconds() -> (seconds since 1Jan1904=w497:timestamp)
      }
    }
    n284 = shared-variable ".\\Variable.lvlib\\stop1"() -> (w425:bool)  [unwired: 1 in, 1 out]
    n285 = shared-variable ".\\Variable.lvlib\\stop2"() -> (w424:bool)  [unwired: 1 in, 1 out]
    n286 = shared-variable ".\\Variable.lvlib\\stop3"() -> (w423:bool)  [unwired: 1 in, 1 out]
    n287 = shared-variable ".\\Variable.lvlib\\stop4"() -> (w422:bool)  [unwired: 1 in, 1 out]
    n288 = case shown="假" w443 {
      tunnel: w447 -> [_ w484]
      tunnel: [FALSE w480] -> w429
      tunnel: [0.0 w479] -> w421
      frame False {
      }
      frame True {
        n289 = shared-variable ".\\Variable.lvlib\\Time 1"() -> (w483:timestamp)  [unwired: 1 in, 1 out]
        n290 = local read "定时 1"() -> (w478:T7)
        n291 = Subtract(x=w484, y=w483) -> (x-y=w482:dbl)
        n292 = Subtract(x=w478, y=w482) -> (x-y=w481:dbl)
        n293 = Round Toward +Infinity(x=w481) -> (ceil(x): smallest int >= x=w479:dbl)
        n294 = Equal To 0?(x=w479) -> (x = 0?=w480:bool)
      }
    }
    n295 = case shown="假" w442 {
      tunnel: w446 -> [_ w472]
      tunnel: [FALSE w471] -> w428
      tunnel: [0.0 w470] -> w420
      frame False {
      }
      frame True {
        n296 = shared-variable ".\\Variable.lvlib\\Time 2"() -> (w474:timestamp)  [unwired: 1 in, 1 out]
        n297 = local read "定时 2"() -> (w469:T7)
        n298 = Subtract(x=w472, y=w474) -> (x-y=w475:dbl)
        n299 = Subtract(x=w469, y=w475) -> (x-y=w473:dbl)
        n300 = Round Toward +Infinity(x=w473) -> (ceil(x): smallest int >= x=w470:dbl)
        n301 = Equal To 0?(x=w470) -> (x = 0?=w471:bool)
      }
    }
    n302 = case shown="真" w441 {
      tunnel: w445 -> [_ w463]
      tunnel: [FALSE w462] -> w427
      tunnel: [0.0 w461] -> w419
      frame False {
      }
      frame True {
        n303 = shared-variable ".\\Variable.lvlib\\Time 3"() -> (w466:timestamp)  [unwired: 1 in, 1 out]
        n304 = local read "定时 3"() -> (w460:T7)
        n305 = Subtract(x=w463, y=w466) -> (x-y=w465:dbl)
        n306 = Subtract(x=w460, y=w465) -> (x-y=w464:dbl)
        n307 = Round Toward +Infinity(x=w464) -> (ceil(x): smallest int >= x=w461:dbl)
        n308 = Equal To 0?(x=w461) -> (x = 0?=w462:bool)
      }
    }
    n309 = case shown="假" w440 {
      tunnel: w444 -> [_ w454]
      tunnel: [FALSE w453] -> w426
      tunnel: [0.0 w452] -> w418
      frame False {
      }
      frame True {
        n310 = shared-variable ".\\Variable.lvlib\\Time 4"() -> (w456:timestamp)  [unwired: 1 in, 1 out]
        n311 = local read "定时 4"() -> (w451:T7)
        n312 = Subtract(x=w454, y=w456) -> (x-y=w457:dbl)
        n313 = Subtract(x=w451, y=w457) -> (x-y=w455:dbl)
        n314 = Round Toward +Infinity(x=w455) -> (ceil(x): smallest int >= x=w452:dbl)
        n315 = Equal To 0?(x=w452) -> (x = 0?=w453:bool)
      }
    }
    n316 = Or(x=w429, y=w425) -> (x .or. y?=w432:bool)
    n317 = Or(x=w427, y=w423) -> (x .or. y?=w431:bool)
    n318 = Or(x=w428, y=w424) -> (x .or. y?=w433:bool)
    n319 = Or(x=w426, y=w422) -> (x .or. y?=w430:bool)
    n320 = case shown="假" w432 {
      selector: w432 -> [_ w496]
      frame False {
      }
      frame True {
        n321 = Not(x=w496) -> (.not. x?=w494:bool)
        n322 = property on="输出 1" class="Bool"("Val(Sgnl)"=w494) -> ()  [unwired: 2 in, 2 out]
        n323 = shared-variable ".\\Variable.lvlib\\order"("tsto1" ("order")) -> ()  [unwired: 1 in, 1 out]
        n324 = property on="停止 1" class="Bool"("Val(Sgnl)"=w494) -> ()  [unwired: 2 in, 2 out]
      }
    }
    n325 = case shown="假" w433 {
      selector: w433 -> [_ w493]
      frame False {
      }
      frame True {
        n326 = Not(x=w493) -> (.not. x?=w491:bool)
        n327 = property on="输出 2" class="Bool"("Val(Sgnl)"=w491) -> ()  [unwired: 2 in, 2 out]
        n328 = shared-variable ".\\Variable.lvlib\\order"("tsto2" ("order")) -> ()  [unwired: 1 in, 1 out]
        n329 = property on="停止 2" class="Bool"("Val(Sgnl)"=w491) -> ()  [unwired: 2 in, 2 out]
      }
    }
    n330 = case shown="真" w431 {
      selector: w431 -> [_ w490]
      frame False {
      }
      frame True {
        n331 = Not(x=w490) -> (.not. x?=w488:bool)
        n332 = property on="输出 3" class="Bool"("Val(Sgnl)"=w488) -> ()  [unwired: 2 in, 2 out]
        n333 = shared-variable ".\\Variable.lvlib\\order"("tsto3" ("order")) -> ()  [unwired: 1 in, 1 out]
        n334 = property on="停止 3" class="Bool"("Val(Sgnl)"=w488) -> ()  [unwired: 2 in, 2 out]
      }
    }
    n335 = case shown="假" w430 {
      selector: w430 -> [_ w487]
      frame False {
      }
      frame True {
        n336 = Not(x=w487) -> (.not. x?=w485:bool)
        n337 = property on="输出 4" class="Bool"("Val(Sgnl)"=w485) -> ()  [unwired: 2 in, 2 out]
        n338 = shared-variable ".\\Variable.lvlib\\order"("tsto4" ("order")) -> ()  [unwired: 1 in, 1 out]
        n339 = property on="停止 4" class="Bool"("Val(Sgnl)"=w485) -> ()  [unwired: 2 in, 2 out]
      }
    }
    n340 = shared-variable ".\\Variable.lvlib\\SetTime 2"(w420) -> ()  [unwired: 1 in, 1 out]
    n341 = shared-variable ".\\Variable.lvlib\\SetTime 3"(w419) -> ()  [unwired: 1 in, 1 out]
    n342 = shared-variable ".\\Variable.lvlib\\SetTime 4"(w418) -> ()  [unwired: 1 in, 1 out]
    n343 = Format Date/Time String(time format string (%c)=w439, seconds (now)=w421, UTC format=w434) -> (date/time string=→"time 1":string)
    n344 = Format Date/Time String(time format string (%c)=w439, seconds (now)=w420, UTC format=w434) -> (date/time string=→"time 2":string)
    n345 = Format Date/Time String(time format string (%c)=w439, seconds (now)=w419, UTC format=w434) -> (date/time string=→"time 3":string)
    n346 = Format Date/Time String(time format string (%c)=w439, seconds (now)=w418, UTC format=w434) -> (date/time string=→"time 4":string)
  }
